vi "getGlyphFile.vi"(8 "error in (no error)":errorcluster, 11 "Categories in":refnum<class "Categories.lvclass">) -> (0 "error out":errorcluster, 2 "Glyph File":string, 3 "Categories out":refnum<class "Categories.lvclass">)   [LabVIEW 2013, in "Categories.lvclass"]
doc: "Dynamic Dispatch VI. Returns the name of the glyph file to be used as a glyph in the tree control. A empty string means no glyph."
uses:
  Categories.lvclass
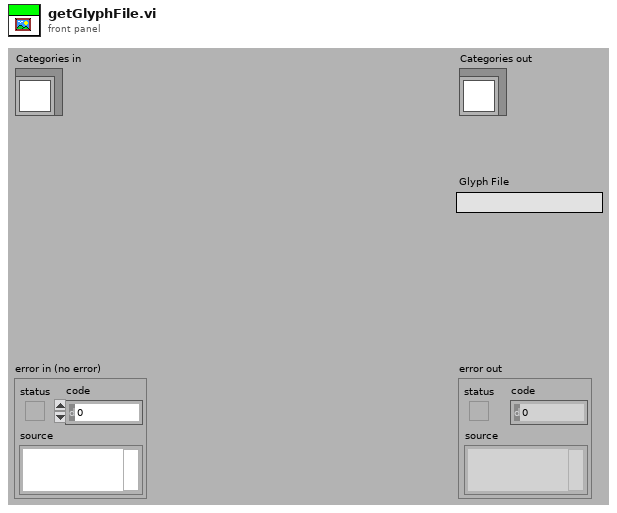
[diagram p1: front panel]
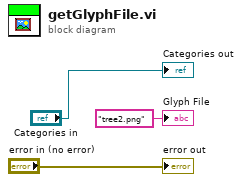
[diagram p0: block diagram]
diagram:
  "error out" <- "error in (no error)"
  "Categories out" <- "Categories in"
  "Glyph File" <- "tree2.png" ("Glyph File")
